vi "auto datalogger user selected.vi"(9 "data log interval (s)":sgl=1.0 min=1, 11 "datalog ref":refnum<file>) -> (0 "File Failure":bool, 3 "File refnum":refnum<file>)   [LabVIEW 2012]
uses:
  DAQ configuration/Sensor buffer command.ctl
  logic buffer cmd.ctl
  calibration/global scale array.vi
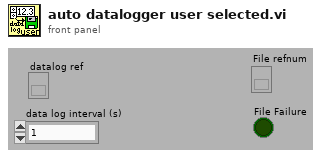
[diagram p1: front panel]
types:
  T1 = typedef "logic buffer cmd.ctl" = enum16{"read", "write ouput settings", "write rules", "write setpoints", "write output descriptions", "write all", "calculate setpoints", "save", "open", "Load all setpoint code", "Load one setpoint code", "Configure one setpoint code"}
  T2 = typedef "Sensor buffer command.ctl" = enum16{"read average", "read recent", "read all", "write", "configure", "clear"}
  T3 = typedef "Sensor data.ctl" = cluster{" Sensor array":T4[], "Time":dbl}
  T4 = typedef "sensor cluster.ctl" = cluster{"voltage":sgl, "scaled":sgl, "units":string, "Out of Range":bool}
  T5 = typedef "variable setpoint.ctl" = cluster{"name":string, "unit":string, "value":dbl, "Type":enum16{"Constant", "Variable"}, "variable":cluster{"selected sensors":i32[], "selected set points":i32[], "VI":path, "Data average interval":T6, "code ref":T7}}
  T6 = typedef "data ave interval.ctl" = dbl
  T7 = typedef "type specifier for control code.ctl" = refnum<vi>
  T8 = typedef "calib array.ctl" = T9[]
  T9 = typedef "conversion.ctl" = cluster{"conversion matrix":sgl[][], "units":string, "name":string, "scale type":T10, "offset (volts)":dbl, "second channel":i8, "correspondence table":T11, "offset (physical units)":dbl, "pH scale":T12, "D.O.":T13}
  T10 = typedef "scale type.ctl" = enum16{"Volts", "Polynomial", "Correspondence Table", "pH", "Dissolved Oxygen", "Quadratic"}
  T11 = typedef "correspondence table.ctl" = cluster{"physical units":dbl, "volts":dbl}[]
  T12 = typedef "pH scale.ctl" = cluster{"Buffers":cluster{"Buffer":dbl, "Calibrated":bool, "V/T":dbl}[], "Temperature":dbl}
  T13 = typedef "DO scale.ctl" = cluster{"Temperature":dbl, "K":dbl, "barometric pressure":dbl}
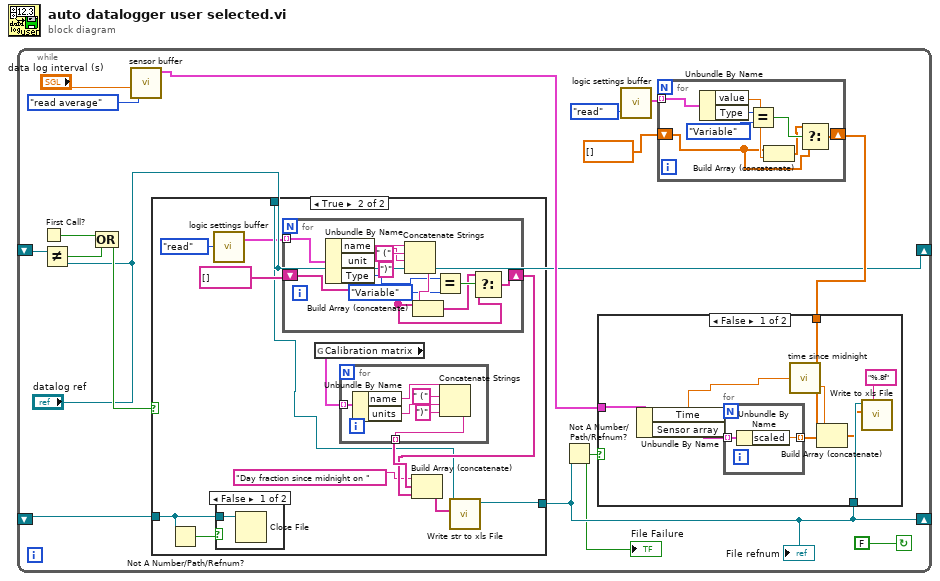
[diagram p0: block diagram]
diagram:
  n1 = while {
    shift-left: _ -> [w16]
    shift-right: ["datalog ref"] -> _
    shift-right: [w12] -> _
    shift-left: _ -> [w11]
    stop <- FALSE continue-if-true
    n2 = First Call?() -> (First Call?: T/F=w14:bool)
    n3 = Not Equal?(x=w16, y="datalog ref") -> (x != y?=w13:bool)
    n4 = Compound Arithmetic op=OR(w14, w13) -> (w10:bool)
    n5 = call "sensor buffer.vi"("command"=Sensor_buffer_command."read average", "smooth interval (s)"="data log interval (s)") -> ("Sensor Data smoothed"=w4:T3)  [unwired: 3 in, 2 out]
    n6 = case shown="True" w10 {
      tunnel: w11 -> [w25 w34]
      tunnel: [w25 w37] -> w12
      tunnel: "datalog ref" -> [_ w29]
      frame False {
      }
      frame True {
        n7 = Not A Number/Path/Refnum?(number/path/refnum=w34) -> (NaN/Path/Refnum?=w33:bool)
        n8 = call "logic settings buffer.vi"("command"=logic_buffer_cmd."read") -> ("Set Points out"=w26:T5[])  [unwired: 11 in, 7 out]
        n9 = case shown="False" w33 {
          tunnel: w34 -> [w50 _]
          frame False {
            n10 = Close File(refnum=w50) -> ()  [unwired: 1 in, 2 out]
          }
          frame True {
          }
        }
        n11 = for {
          tunnel: w26 -> [w49] mode=indexing
          shift-right: [w38] -> w30
          shift-left: string[] [] -> [w39]
          n12 = Unbundle By Name(w49) -> ("name"=w46:string, "unit"=w45:string, "Type"=w42:enum16{"Constant", "Variable"})
          n13 = Concatenate Strings(w46, " (" ("Substring"), w45, ")" ("Substring")) -> (w43:string)
          n14 = Build Array (concatenate)(w39, w43) -> (w40:string[])
          n15 = Equal?(x=w42, y=enum16{"Constant", "Variable"}."Variable") -> (x = y?=w44:bool)
          n16 = Select(t=w40, s=w44, f=w39) -> (s? t:f=w38:string[])
        }
        n17 = global read "global scale array.vi" "Calibration matrix"() -> (w36:T8)
        n18 = for {
          tunnel: w36 -> [w56] mode=indexing
          tunnel: [w51] -> w35 mode=indexing
          n19 = Unbundle By Name(w56) -> ("name"=w55:string, "units"=w53:string)
          n20 = Concatenate Strings(w55, " (" ("Substring"), w53, ")" ("Substring")) -> (w51:string)
        }
        n21 = Build Array (concatenate)("Day fraction since midnight on " ("Substring"), w35, w30) -> (w27:string[])
        n22 = call "Write str to xls File.vi"("1D data"=w27, "refnum"=w29) -> ("dup refnum"=w37:refnum<file>)  [unwired: 8 in, 1 out]
      }
    }
    "File refnum" <- w12
    n23 = Not A Number/Path/Refnum?(number/path/refnum=w12) -> (NaN/Path/Refnum?=w9:bool)
    "File Failure" <- w9
    n24 = call "logic settings buffer.vi"("command"=logic_buffer_cmd."read") -> ("Set Points out"=w5:T5[])  [unwired: 11 in, 7 out]
    n25 = for {
      tunnel: w5 -> [w24] mode=indexing
      shift-right: [w18] -> w2
      shift-left: dbl[] [] -> [w17]
      n26 = Unbundle By Name(w24) -> ("value"=w20:dbl, "Type"=w23:enum16{"Constant", "Variable"})
      n27 = Equal?(x=w23, y=enum16{"Constant", "Variable"}."Variable") -> (x = y?=w21:bool)
      n28 = Build Array (concatenate)(w17, w20) -> (w19:dbl[])
      n29 = Select(t=w19, s=w21, f=w17) -> (s? t:f=w18:dbl[])
    }
    n30 = case shown="False" w9 {
      tunnel: w12 -> [w62 _]
      tunnel: w4 -> [w59 _]
      tunnel: w2 -> [w58 _]
      frame False {
        n31 = Unbundle By Name(w59) -> ("Time"=w61:dbl, "Sensor array"=w64:T4[])
        n32 = for {
          tunnel: w64 -> [w67] mode=indexing
          tunnel: [w66] -> w63 mode=indexing
          n33 = Unbundle By Name(w67) -> ("scaled"=w66:sgl)
        }
        n34 = call "time since midnight.vi"("seconds since 1Jan1904"=w61) -> ("Days"=w60:dbl)  [unwired: 1 out]
        n35 = Build Array (concatenate)(w60, w63, w58) -> (w57:dbl[])
        n36 = call "Write to xls File.vi"("format (%.3f)"="%.8f", "1D data"=w57, "refnum"=w62) -> ()  [unwired: 7 in, 2 out]
      }
      frame True {
      }
    }
  }
